vi "Create.vi"(8 "error in (no error)":errorcluster, 10 "Comparator":refnum<class "Comparator.lvclass">) -> (0 "error out":errorcluster, 3 "One":refnum<class "One.lvclass">)   [LabVIEW 2020, in "One.lvlib" / "One.lvclass"]
uses:
  One.lvclass
  Core/Comparator/Comparator.lvclass
  One.lvclass/One.ctl
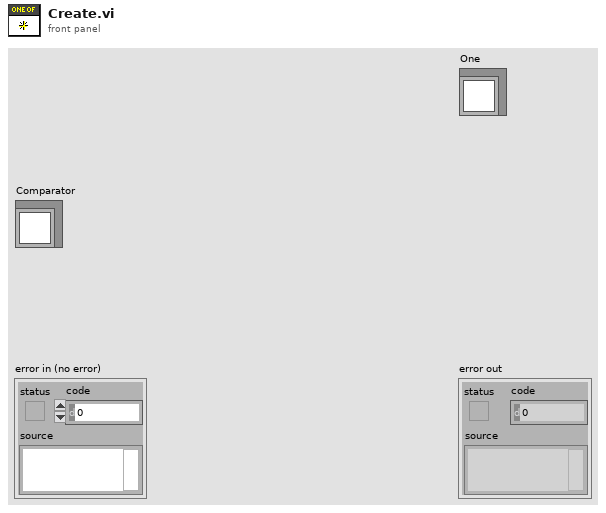
[diagram p1: front panel]
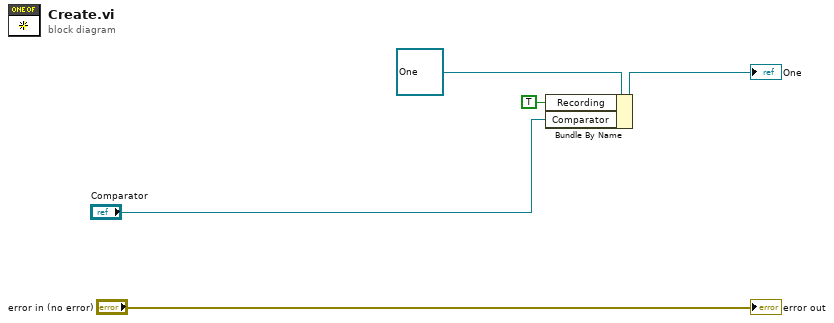
[diagram p0: block diagram]
diagram:
  n1 = Bundle By Name(cluster=refnum<class "One.lvclass"> refnum ("One"), "Recording"=TRUE, "Comparator"="Comparator") -> (→"One":refnum<class "One.lvclass">)
  "error out" <- "error in (no error)"
